vi "Pre Launch Init.vi"(11 "Post Analysis in":refnum<class "Post Analysis.lvclass">) -> (0 "error out":errorcluster, 3 "Post Analysis out":refnum<class "Post Analysis.lvclass">)   [LabVIEW 2023, in "Data Analysis.lvlib" / "Post Analysis.lvlib" / "Post Analysis.lvclass"]
doc: "(<B>Filename</B>: Actor Framework.lvlib:Actor.lvclass:Pre Launch Init.vi)\n\nDefines behavior that occurs after the Launch Nested Actor method is invoked but before the actor's Actor Core method begins running.\n\nBy default, this method does nothing. A descendant class may override it to define behavior."
uses:
  Post Analysis.lvclass
  HardwareAbstractionLayer_LVOOP/Database/SQL Public VI/Control/DB Options.ctl
  <vilib>/ActorFramework/Actor/Actor.lvclass
  HardwareAbstractionLayer_LVOOP/Database/Database.lvclass
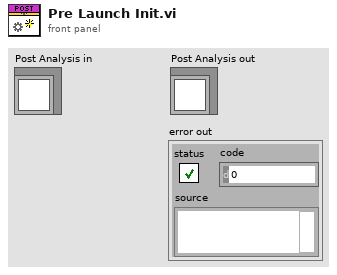
[diagram p1: front panel]
types:
  T1 = typedef "HardwareAbstractionLayer_LVOOP.lvlib/Database.lvclass/DB Options.ctl" = enum16{"Init", "Select Data", "Insert Data", "Update Data", "Delete Data", "Execute Query", "Create Schema", "Create Table", "List Tables", "List Columns", "Close"}
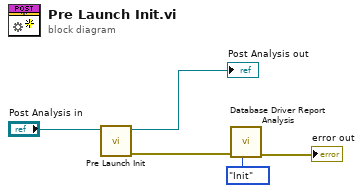
[diagram p0: block diagram]
diagram:
  n1 = call-parent "Pre Launch Init.vi"("Actor in"="Post Analysis in") -> ("error out"=w2:errorcluster, "Actor out"=→"Post Analysis out":refnum<class "Post Analysis.lvclass">)  [unwired: 9 in]
  n2 = call "Database Driver Report Analysis.vi"("Options"=DB_Options."Init", "error in"=w2) -> ("error out"=→"error out":errorcluster)  [unwired: 6 in, 3 out]
